vi "_Remote Get RT Status.vi"(0 "RT Ready":bool, 1 "error in (no error)":errorcluster) -> (2 "InstrState":T1, 3 "RT Ready Out":bool, 4 "StatusIndicator":u16(ring)=1 caption="Status Indicator")   [LabVIEW 2018]
uses:
  Type/_RT Instrument State.ctl
  Type/_RT Command.ctl
  Configuration/_Global Configuration.vi
  <vilib>/Utility/config.llb/Read Key (String).vi
  <vilib>/Utility/config.llb/NI_LVConfig.lvlib
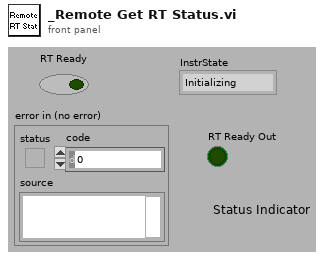
[diagram p1: front panel]
types:
  T1 = typedef "_RT Instrument State.ctl" = enum16{"Initializing", "Mass Spectrometer is Off", "Starting Up", "Turning Power Off", "Going to Standby", "Roughing Pump Ready", "Turning Turbo Off", "Turbo Startup", "Turbopump Ready", "Checking Vacuum", "Going to Ready", "Ready", "Running", "Source Standby", "Lost Communication", "Shutting Down", "Fault", "24V Standby", "Go to 24V Standby", "Turbopump Ready-Waiting"}
  T2 = typedef "_RT Command.ctl" = enum16{"xml Start Run", "xml Start Actual Run", "xml Stop Run", "xml Runtime Update", "xml Get Status", "xml Get Table", "xml Set Table", "xml Get Configuration", "xml System Status", "xml Set LC Input Logic", "xml Get Data", "xml Get Info", "Start", "StartActualRun", "Stop", "Runtime Update", "Get Data", "Get Info", "Get Status", "Get Param", "Get Config", "Get Table", "Read ADC", "Set Oscillator", "Update Config", "Update Table", "Set All Pol", "Set Pol and DC", "Set Max Mass", "Toggle RP", "Toggle EL", "Set PIC", "Initialize Turbo", "Send Turbo Comm", "Close Turbo", "P1", "P2", "P3", "Send Serial", "Set LC Out", "Get LC In", "Read VAC", "Test Table", "Toggle Power", "Get Startup", "Set Startup", "Get ADC Table", "Set ADC Table", "Get Brief Status", "Get Detail Status", "Auxiliary Update", "Set CC Logics", "Test Channel", "Set CC Input Logics", "Ignore Error", "invalid"}
  T3 = typedef "NI_LVConfig.lvlib/Config Data RefNum.ctl" = refnum<k1>
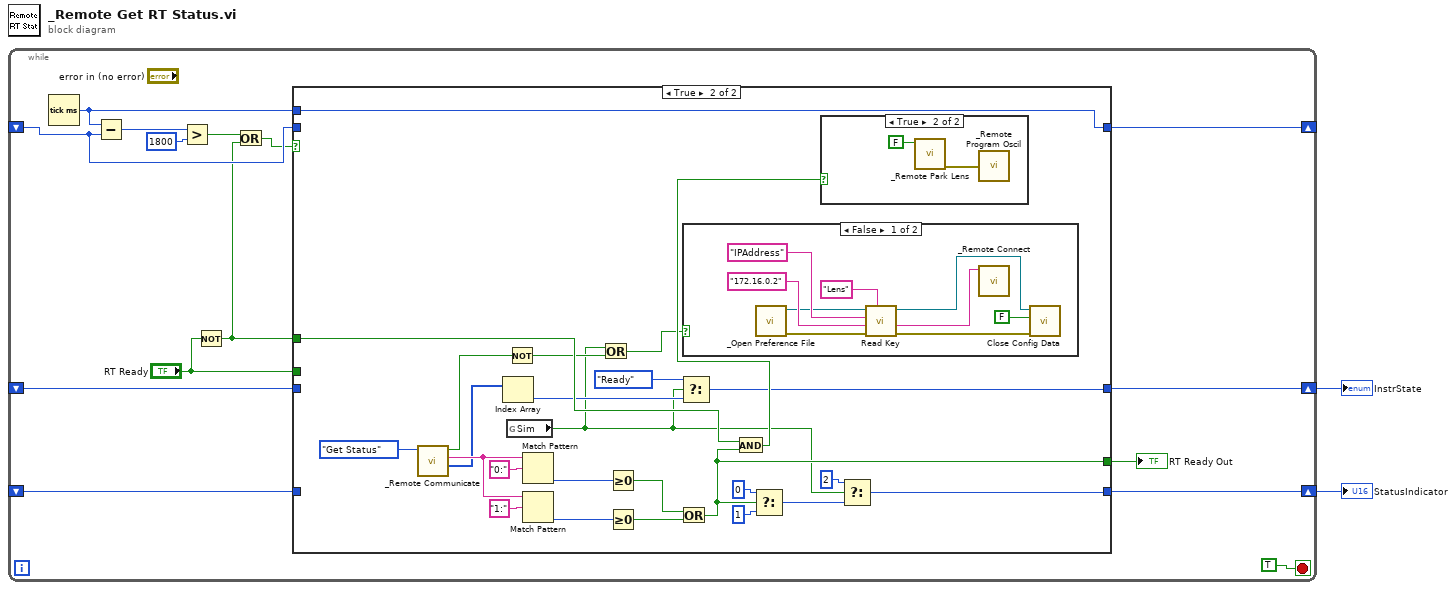
[diagram p0: block diagram]
diagram:
  n1 = while {
    shift-right: [w15] -> _
    shift-left: _ -> [w12]
    shift-right: [w6] -> w2
    shift-left: _ -> [w5]
    shift-right: [w4] -> w1
    shift-left: _ -> [w3]
    stop <- TRUE stop-if-true
    n2 = Tick Count (ms)() -> (millisecond timer value=w16:u32)
    n3 = Subtract(x=w16, y=w12) -> (x-y=w14:u32)
    n4 = Greater?(x=w14, y=u32 1800) -> (0:w10:bool)
    n5 = Not(x="RT Ready") -> (.not. x?=w11:bool)
    n6 = Or(x=w10, y=w11) -> (x .or. y?=w9:bool)
    n7 = case shown="True" w9 {
      tunnel: w11 -> [_ w40]
      tunnel: [w21 w36] -> w15
      tunnel: w16 -> [_ w36]
      tunnel: w12 -> [w21 _]
      tunnel: [w20 w26] -> w8
      tunnel: "RT Ready" -> [w20 _]
      tunnel: [w19 w32] -> w6
      tunnel: w5 -> [w19 _]
      tunnel: [w18 w22] -> w4
      tunnel: w3 -> [w18 _]
      frame False {
      }
      frame True {
        n8 = call "_Remote Communicate.vi"("Command"=_RT_Command."Get Status") -> ("Data Array"=w35:i32[], "Info"=w41:string, "CommErr"=w29:bool)  [unwired: 5 in, 1 out]
        n9 = Index Array(array=w35) -> (element=w34:i32)  [unwired: 1 in]
        n10 = Not(x=w29) -> (.not. x?=w31:bool)
        n11 = global read "_Global Configuration.vi" "Sim"() -> (w24:bool)
        n12 = Match Pattern(string=w41, regular expression="0:") -> (offset past match=w45:i32)  [unwired: 4 out]
        n13 = Match Pattern(string=w41, regular expression="1:") -> (offset past match=w42:i32)  [unwired: 4 out]
        n14 = Or(x=w24, y=w31) -> (x .or. y?=w30:bool)
        n15 = Greater Or Equal To 0?(x=w45) -> (x >= 0?=w38:bool)
        n16 = Greater Or Equal To 0?(x=w42) -> (x >= 0?=w37:bool)
        n17 = Or(x=w38, y=w37) -> (x .or. y?=w26:bool)
        n18 = Select(t=_RT_Instrument_State."Ready" ("InstrState"), s=w24, f=w34) -> (s? t:f=w32:i32)
        n19 = case shown="False" w30 {
          frame False {
            n20 = call "_Open Preference File.vi"() -> ("error"=w47:errorcluster, "refnum"=w48:T3)  [unwired: 3 in, 3 out]
            n21 = call-poly <vilib>:"Read Key.vi"("section"="Lens", "error in (no error)"=w47, "default value"="172.16.0.2", "key"="IPAddress" ("section"), "refnum"=w48) -> ("error out"=w51:errorcluster, "value"=w49:string, "refnum out"=w52:T3)  [unwired: 1 in, 3 out]
            n22 = call "_Remote Connect.vi"("IP Address"=w49) -> ()  [unwired: 1 in, 6 out]
            n23 = call <vilib>:"Close Config Data.vi"("error in (no error)"=w51, "write file if changed (T)"=FALSE ("write configuration file? (T)"), "refnum"=w52) -> ()  [unwired: 9 out]
          }
          frame True {
          }
        }
        n24 = And(x=w40, y=w26) -> (x .and. y?=w39:bool)
        n25 = Select(t=u16 0 ("LC Connection"), s=w26, f=u16 1 ("LC Connection")) -> (s? t:f=w23:u16)
        n26 = case shown="True" w39 {
          frame False {
          }
          frame True {
            n27 = call "_Remote Park Lens.vi"("All Ch (F)"=FALSE) -> ("error out"=w56:errorcluster)  [unwired: 1 in, 5 out]
            n28 = call "_Remote Program Oscil.vi"("error in (no error)"=w56) -> ()  [unwired: 1 out]
          }
        }
        n29 = Select(t=u16 2 ("LC Connection"), s=w24, f=w23) -> (s? t:f=w22:u16)
      }
    }
    "RT Ready Out" <- w8
  }
  "InstrState" <- w2
  "StatusIndicator" <- w1
